vi "旋转函数.vi"(10 "原始方块位置":i32[][](array[numeric])) -> (0 "旋转方块位置":i32[][](array[numeric]), 2 "旋转后随机方块":bool[][](array[boolean]))   [LabVIEW 2013]
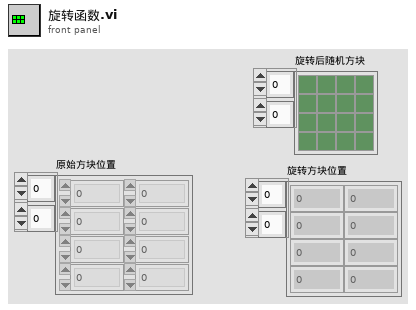
[diagram p1: front panel]
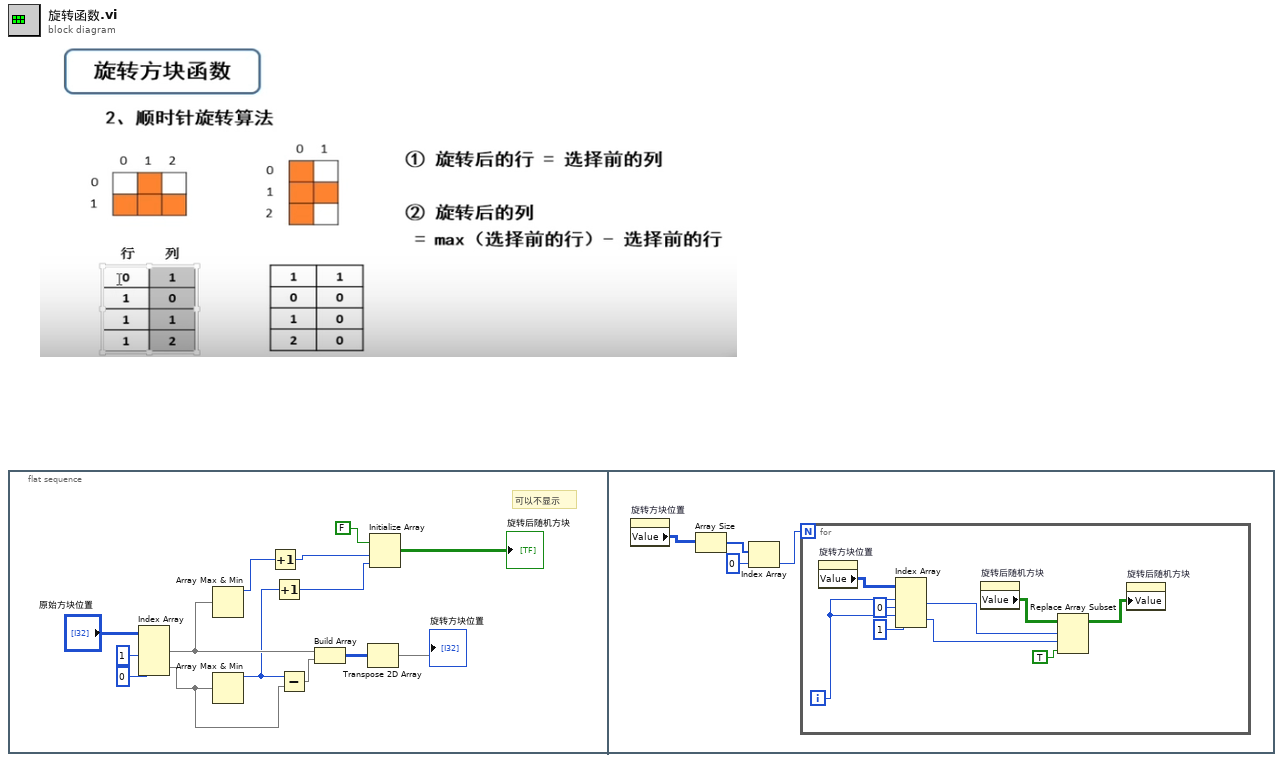
[diagram p0: block diagram]
diagram:
  n1 = flat-sequence {
    frame #0 {
      # "可以不显示"
      n2 = Index Array(array="原始方块位置", index (col) #1=1 ("禁用的索引 (列)"), index (col) #2=0 ("索引 (列)")) -> (element #1=w7:i32[], element #2=w11:i32[])  [unwired: 2 in]
      n3 = Array Max & Min(array=w7) -> (max value=w6:i32)  [unwired: 3 out]
      n4 = Array Max & Min(array=w11) -> (max value=w5:i32)  [unwired: 3 out]
      n5 = Increment(x=w6) -> (x+1=w3:i32)
      n6 = Increment(x=w5) -> (x+1=w4:i32)
      n7 = Subtract(x=w5, y=w11) -> (x-y=w10:i32[])
      n8 = Build Array(w7, w10) -> (w9:i32[][])
      n9 = Transpose 2D Array(2D array=w9) -> (transposed array=→"旋转方块位置":i32[][])
      n10 = Initialize Array(FALSE, w3, w4) -> (→"旋转后随机方块":bool[][])
    }
    frame #1 {
      n11 = property on="旋转方块位置" class="Arr (严格)"() -> ("Value"=w16:i32[][])  [unwired: 2 in, 2 out]
      n12 = Array Size(array=w16) -> (size(s)=w15:i32[])
      n13 = Index Array(array=w15, index=0 ("索引")) -> (element=w17:i32)
      n14 = for {
        N: w17 -> [_]
        i -> [w26]
        n15 = property on="旋转方块位置" class="Arr (严格)"() -> ("Value"=w27:i32[][])  [unwired: 2 in, 2 out]
        n16 = Index Array(array=w27, index (row) #1=w26, index (col) #1=0 ("禁用的索引 (列)"), index (row) #2=w26, index (col) #2=1 ("禁用的索引 (列)")) -> (element #1=w22:i32, element #2=w21:i32)
        n17 = property on="旋转后随机方块" class="Arr (严格)"() -> ("Value"=w23:bool[][])  [unwired: 2 in, 2 out]
        n18 = Replace Array Subset(array=w23, new element=TRUE, index (row)=w22, index (col)=w21) -> (w20:bool[][])
        n19 = property on="旋转后随机方块" class="Arr (严格)"("Value"=w20) -> ()  [unwired: 2 in, 2 out]
      }
    }
  }
